vi "Get Item List from JSON File.vi"(8 "error in (no error)":errorcluster, 11 "Byte Stream File in":refnum<file>) -> (0 "error out":errorcluster, 1 "JSON String":string, 2 "Item List":string[](array[string]), 3 "Byte Stream File out":refnum<file>)   [LabVIEW 2020, in "JSON File Manipulation.lvlib"]
doc: "Reads the JSON file and returns the List of Items based on the Item Path input."
uses:
  JSON File Manipulation.lvlib
  <vilib>/JDP Science/JSONtext/String Subset.vi
  <vilib>/JDP Science/JSONtext/support/Strip Quotes and Unescape.vi
  <vilib>/JDP Science/JSONtext/Parsing/Parse Full Path or Item Name.vi
  <vilib>/JDP Science/JSONtext/Offset/Find Item Locations by Path.vi
  <vilib>/JDP Science/JSONtext/support/Unescape JSON string.vi
  <vilib>/JDP Science/JSONtext/JSONtext.lvlib
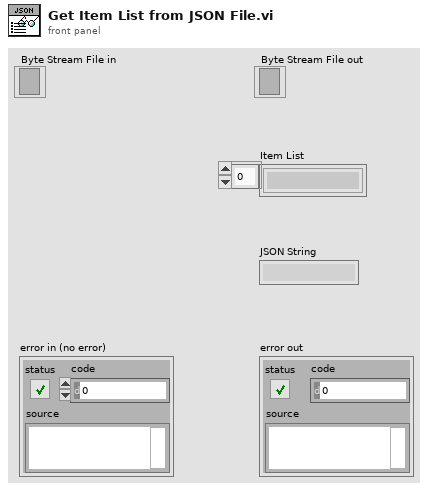
[diagram p1: front panel]
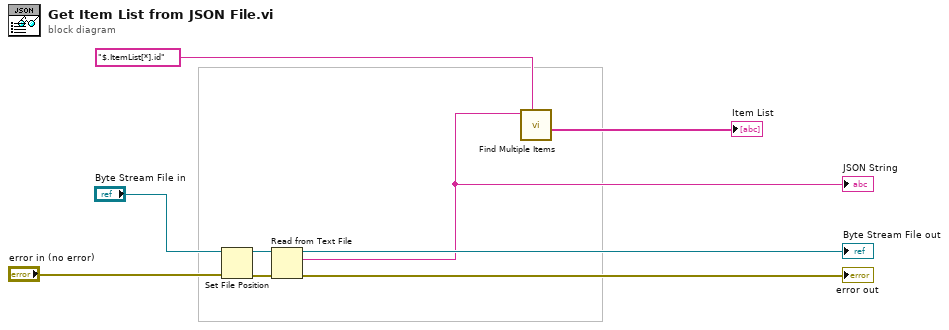
[diagram p0: block diagram]
diagram:
  n1 = Set File Position(refnum="Byte Stream File in", error in="error in (no error)") -> (refnum out=w8:refnum<file>, error out=w6:errorcluster)  [unwired: 2 in]
  n2 = Read from Text File(file (use dialog)=w8, error in=w6) -> (refnum out=→"Byte Stream File out":refnum<file>, text=w3:string, error out=→"error out":errorcluster)  [unwired: 2 in, 1 out]
  "JSON String" <- w3
  n3 = call <vilib>:"Find Multiple Items.vi"("$Path or Item Name"="$.ItemList[*].id", "JSON"=w3) -> ("<JSON>"=→"Item List":string[])  [unwired: 6 in, 3 out]
